vi "Test.vi"() -> ()   [LabVIEW 2015]
uses:
  <vilib>/rvi/Analysis/control/PID/Typedef/niFpgaPID_PIGains.ctl
  <vilib>/rvi/Analysis/control/PID/SubVIs/niFpgaPID_PIWrapper.vi
panel:
  in  "I":i16
  in  "P":i16
  in  "X":i16
  out "output":i16
  in  "setpoint":i16
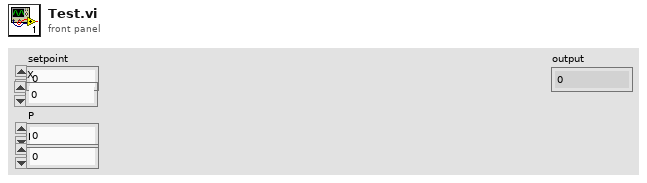
[diagram p1: front panel]
types:
  T1 = typedef "niFpgaPID_PIGains.ctl" = cluster{"proportional gain":sgl, "integral gain":sgl}
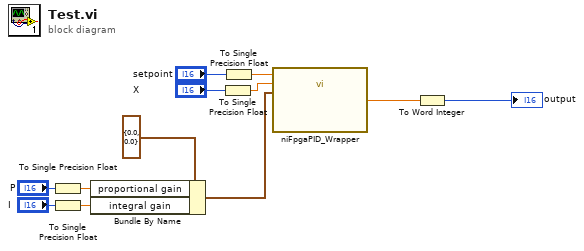
[diagram p0: block diagram]
diagram:
  n1 = To Single Precision Float(number="P") -> (single precision float=w4:sgl)
  n2 = To Single Precision Float(number="I") -> (single precision float=w2:sgl)
  n3 = Bundle By Name(cluster=T1 {"proportional gain"=0.0, "integral gain"=0.0} ("gains"), "proportional gain"=w4, "integral gain"=w2) -> (w1:T1)
  n4 = To Single Precision Float(number="X") -> (single precision float=w7:sgl)
  n5 = To Single Precision Float(number="setpoint") -> (single precision float=w11:sgl)
  n6 = call-poly <vilib>:"niFpgaPID_Wrapper.vi"("setpoint"=w11, "process variable"=w7, "gains"=w1) -> ("output"=w10:sgl)  [unwired: 10 in, 2 out]
  n7 = To Word Integer(number=w10) -> (16bit integer=→"output":i16)
